vi "BrowseTDMSFile.vi"() -> (1 "No files":bool=TRUE, 3 "Selected traces":string[](array[string]))   [LabVIEW 2018]
uses:
  <vilib>/gmath/statdist.llb/st_Percentiles (scalar).vi
  <vilib>/gmath/NI_Gmath.lvlib
panel:
  in  "Deselect all":bool
  out "ScanCode":i16
  in  "Cancel":bool
  in  "Change file":bool
  in  "Sort":bool
  out "F(z)":cluster{"Data":dbl[], "Data":dbl[]}[](graph)
  in  "Select trace":u16(ring)=65535 items=["C:\\Users\\tweezer_user\\Data\\211221\\data_004.tdms: 58", "C:\\Users\\tweezer_user\\Data\\211221\\data_004.tdms: 0", "C:\\Users\\tweezer_user\\Data\\211221\\data_004.tdms: 2", "C:\\Users\\tweezer_user\\Data\\211221\\data_004.tdms: 30", "C:\\Users\\tweezer_user\\Data\\211221\\data_004.tdms: 44", "C:\\Users\\tweezer_user\\Data\\211221\\data_004.tdms: 55", "C:\\Users\\tweezer_user\\Data\\211221\\data_004.tdms: 41", "C:\\Users\\tweezer_user\\Data\\211221\\data_004.tdms: 22", "C:\\Users\\tweezer_user\\Data\\211221\\data_004.tdms: 48", "C:\\Users\\tweezer_user\\Data\\211221\\data_004.tdms: 21", "C:\\Users\\tweezer_user\\Data\\211221\\data_004.tdms: 24", "C:\\Users\\tweezer_user\\Data\\211221\\data_004.tdms: 54", "C:\\Users\\tweezer_user\\Data\\211221\\data_004.tdms: 1", "C:\\Users\\tweezer_user\\Data\\211221\\data_004.tdms: 3", "C:\\Users\\tweezer_user\\Data\\211221\\data_004.tdms: 11", "C:\\Users\\tweezer_user\\Data\\211221\\data_004.tdms: 39", "C:\\Users\\tweezer_user\\Data\\211221\\data_004.tdms: 25", "C:\\Users\\tweezer_user\\Data\\211221\\data_004.tdms: 45", "C:\\Users\\tweezer_user\\Data\\211221\\data_004.tdms: 37", "C:\\Users\\tweezer_user\\Data\\211221\\data_004.tdms: 38", "C:\\Users\\tweezer_user\\Data\\211221\\data_004.tdms: 43", "C:\\Users\\tweezer_user\\Data\\211221\\data_004.tdms: 50", "C:\\Users\\tweezer_user\\Data\\211221\\data_004.tdms: 10", "C:\\Users\\tweezer_user\\Data\\211221\\data_004.tdms: 42", "C:\\Users\\tweezer_user\\Data\\211221\\data_004.tdms: 4", "C:\\Users\\tweezer_user\\Data\\211221\\data_004.tdms: 23", "C:\\Users\\tweezer_user\\Data\\211221\\data_004.tdms: 34", "C:\\Users\\tweezer_user\\Data\\211221\\data_004.tdms: 32", "C:\\Users\\tweezer_user\\Data\\211221\\data_004.tdms: 28", "C:\\Users\\tweezer_user\\Data\\211221\\data_004.tdms: 31", "C:\\Users\\tweezer_user\\Data\\211221\\data_004.tdms: 33", "C:\\Users\\tweezer_user\\Data\\211221\\data_004.tdms: 35", "C:\\Users\\tweezer_user\\Data\\211221\\data_004.tdms: 6", "C:\\Users\\tweezer_user\\Data\\211221\\data_004.tdms: 18", "C:\\Users\\tweezer_user\\Data\\211221\\data_004.tdms: 19", "C:\\Users\\tweezer_user\\Data\\211221\\data_004.tdms: 36", "C:\\Users\\tweezer_user\\Data\\211221\\data_004.tdms: 29", "C:\\Users\\tweezer_user\\Data\\211221\\data_004.tdms: 53", "C:\\Users\\tweezer_user\\Data\\211221\\data_004.tdms: 57", "C:\\Users\\tweezer_user\\Data\\211221\\data_004.tdms: 20", "C:\\Users\\tweezer_user\\Data\\211221\\data_004.tdms: 7", "C:\\Users\\tweezer_user\\Data\\211221\\data_004.tdms: 56", "C:\\Users\\tweezer_user\\Data\\211221\\data_004.tdms: 47", "C:\\Users\\tweezer_user\\Data\\211221\\data_004.tdms: 51", "C:\\Users\\tweezer_user\\Data\\211221\\data_004.tdms: 49", "C:\\Users\\tweezer_user\\Data\\211221\\data_004.tdms: 9", "C:\\Users\\tweezer_user\\Data\\211221\\data_004.tdms: 8", "C:\\Users\\tweezer_user\\Data\\211221\\data_004.tdms: 12", "C:\\Users\\tweezer_user\\Data\\211221\\data_004.tdms: 5", "C:\\Users\\tweezer_user\\Data\\211221\\data_004.tdms: 14", "C:\\Users\\tweezer_user\\Data\\211221\\data_004.tdms: 40", "C:\\Users\\tweezer_user\\Data\\211221\\data_004.tdms: 27", "C:\\Users\\tweezer_user\\Data\\211221\\data_004.tdms: 46", "C:\\Users\\tweezer_user\\Data\\211221\\data_004.tdms: 13", "C:\\Users\\tweezer_user\\Data\\211221\\data_004.tdms: 16", "C:\\Users\\tweezer_user\\Data\\211221\\data_004.tdms: 15", "C:\\Users\\tweezer_user\\Data\\211221\\data_004.tdms: 52", "C:\\Users\\tweezer_user\\Data\\211221\\data_004.tdms: 17", "C:\\Users\\tweezer_user\\Data\\211221\\data_004.tdms: 26", "C:\\Users\\tweezer_user\\Data\\211221\\data_004.tdms: 473"]
  in  "OK":bool
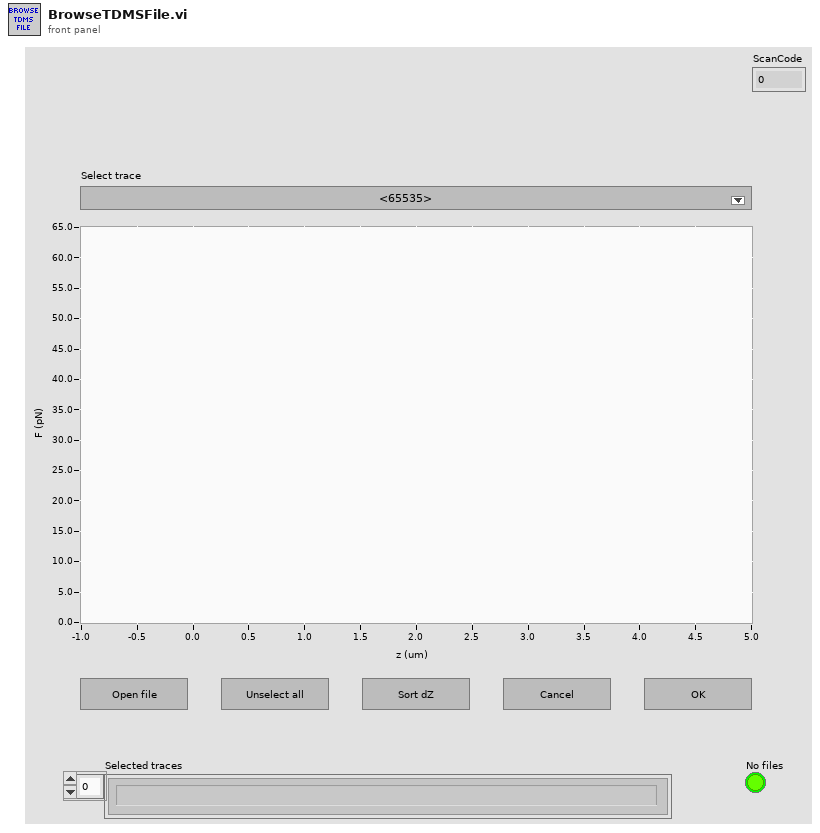
[diagram p1: front panel]
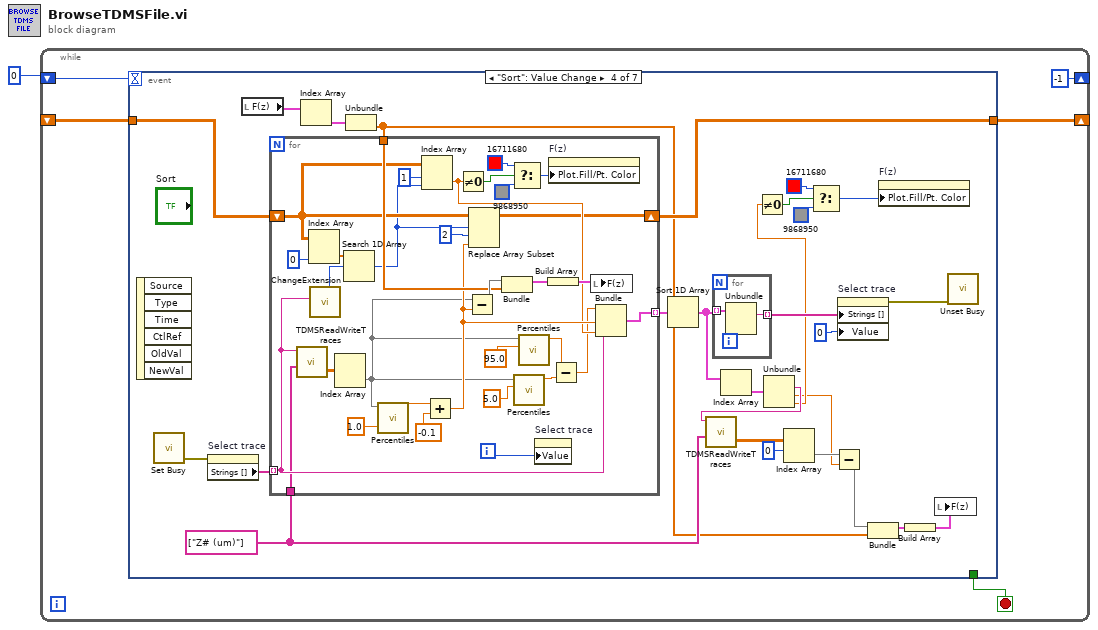
[diagram p0: block diagram]
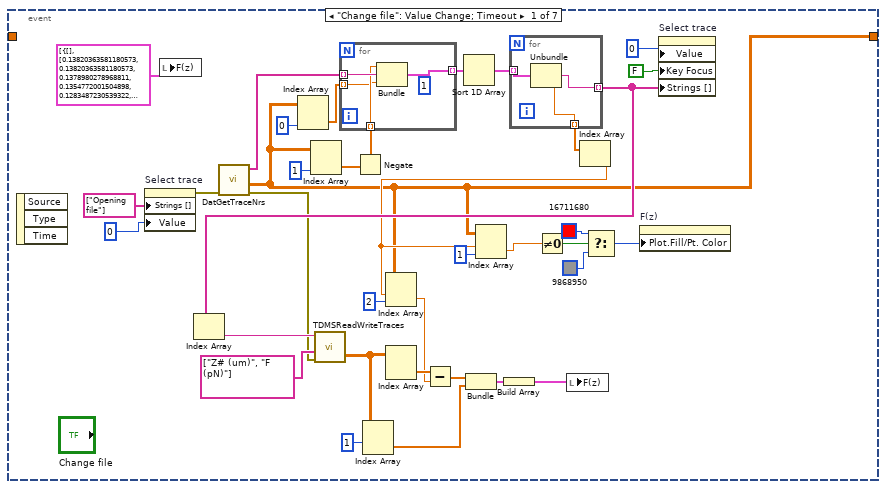
[diagram p2: hidden frame]
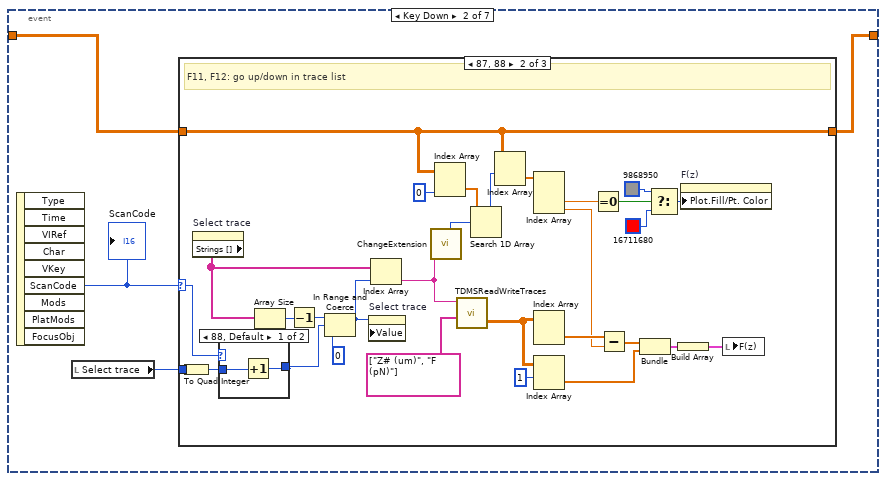
[diagram p3: hidden frame]
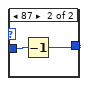
[diagram p5: hidden frame]
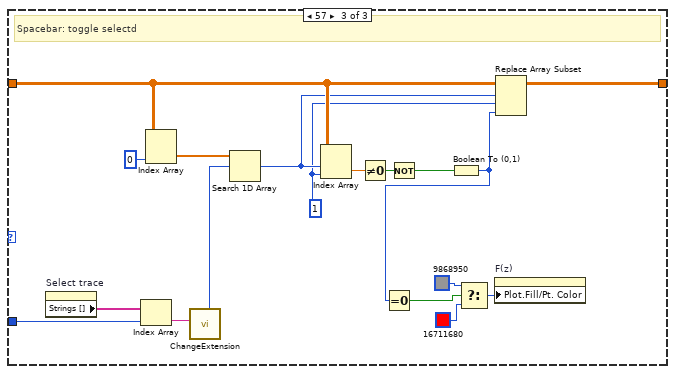
[diagram p6: hidden frame]
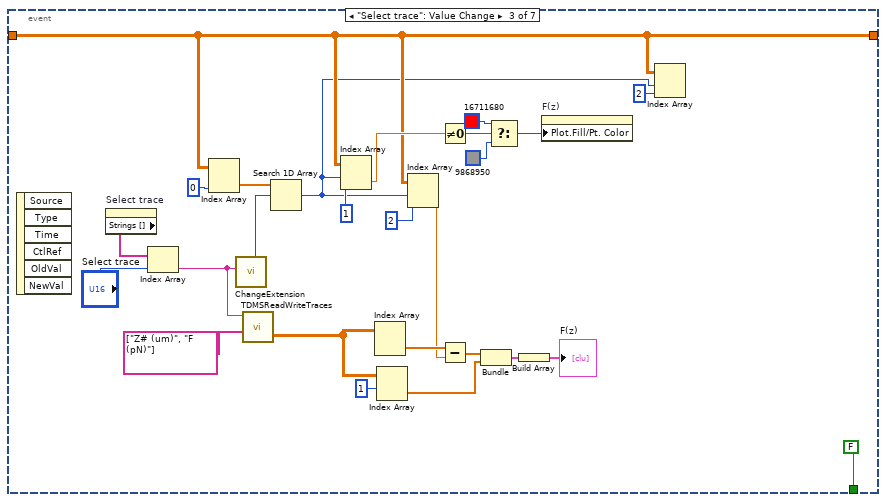
[diagram p7: hidden frame]
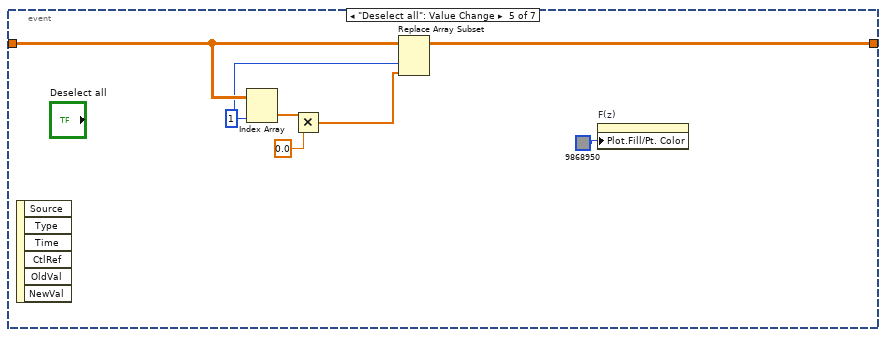
[diagram p8: hidden frame]
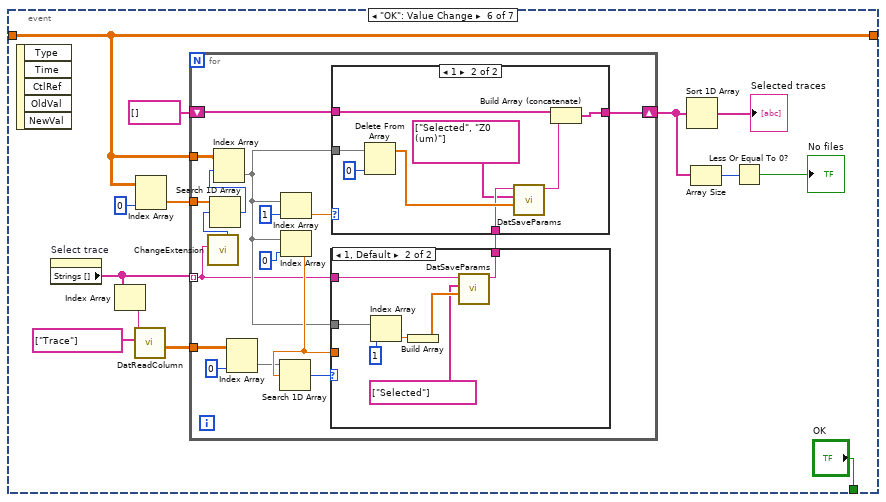
[diagram p9: hidden frame]
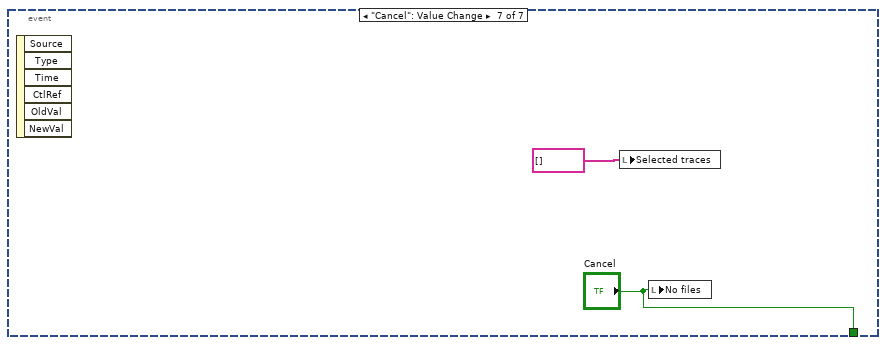
[diagram p12: hidden frame]
diagram:
  n1 = while {
    shift-right: [-1 ("Listbox")] -> _
    shift-left: 0 ("Listbox") -> [w5]
    shift-right: [w2] -> _
    shift-left: _ -> [w3]
    stop <- w6 stop-if-true
    n2 = event shown="[3] \"Sort\": Value Change" {
      selector: _ -> [_ _ _ _ _ _ _]
      dyn-events: _ -> [_ _ _ _ _ _ _]
      timeout: w5 -> [_ _ _ _ _ _ _]
      tunnel: [_ _ FALSE ("stop") _ _ "OK" "Cancel"] -> w6
      tunnel: [w10 w51 w109 w153 w195 w201 _] -> w2
      tunnel: w3 -> [_ w52 w109 w154 w198 w201 _]
      event "Change file": Value Change; Timeout {
        n3 = event-data() -> ()  [unwired: 1 in, 3 out]
        n4 = property on="Select trace" class="Ring (strict)"("Strings []"=string[] ["Opening file"], "Value"=0 ("Top Row")) -> (error out=w23:errorcluster)  [unwired: 2 in, 1 out]
        n5 = local write "F(z)"(cluster{"Data":i32[], "Data":dbl[]}[] [{"Data"=[], "Data"=[0.13820363581180573, 0.13820363581180573, 0.1378980278968811, 0.1354772001504898, 0.1283487230539322, 0.12796370685100555, 0.12760481238365173, 0.12726476788520813, 0.126942977309227, 0.12663885951042175, 0.12635183334350586, 0.12608134746551514, 0.12582682073116302, 0.12558774650096893, 0.1253635585308075, 0.12515376508235931, 0.12495782971382141, 0.1247752457857132, 0.12460550665855408, 0.12444813549518585, 0.12430262565612793, 0.1241685003042221, 0.12404527515172958, 0.12393248826265335, 0.12382965534925461, 0.12373632192611694, 0.12365201860666275, 0.12357629835605621, 0.12350869178771973, 0.12344875186681747, 0.12339602410793304, 0.12335006892681122, 0.12331042438745499, 0.12327665835618973, 0.12324832379817963, 0.12322498112916946, 0.12320617586374283, 0.1231914833188057, 0.12318044900894165, 0.12317264080047607, 0.12316761910915375, 0.12316494435071945, 0.12316489964723587, 0.12408066540956497, 0.12665148079395294, 0.13009892404079437, 0.13340164721012115, 0.1366782933473587, 0.1401367038488388, 0.1436801254749298, 0.14730530977249146, 0.15101973712444305, 0.15482020378112793, 0.15873165428638458, 0.16275079548358917, 0.16688737273216248, 0.17111752927303314, 0.17530791461467743, 0.17975105345249176, 0.1843348741531372, 0.1890215128660202, 0.19384075701236725, 0.19893240928649902, 0.20381732285022736, 0.20893964171409607, 0.21432308852672577, 0.21960188448429108, 0.22516034543514252, 0.23087568581104279, 0.2368132770061493, 0.2428968846797943, 0.24884368479251862, 0.25512930750846863, 0.26159971952438354, 0.268232524394989, 0.2750486135482788, 0.2820947766304016, 0.2891634702682495, 0.296439528465271, 0.3039502501487732, 0.3116407096385956, 0.31944137811660767, 0.32760921120643616, 0.3358848989009857, 0.34432253241539, 0.3531827926635742, 0.3622758090496063, 0.3714924454689026, 0.3809875249862671, 0.39067110419273376, 0.4001978039741516, 0.4104802906513214, 0.42095404863357544, 0.43167173862457275, 0.44273218512535095, 0.45405450463294983, 0.4653382897377014, 0.47709932923316956, 0.4893254041671753, 0.5018249154090881, 0.5145537853240967, 0.5275917649269104, 0.541254997253418, 0.5551921725273132, 0.5689001679420471, 0.5834644436836243, 0.5981636643409729, 0.6131883263587952, 0.6288307309150696, 0.645302414894104, 0.6615437865257263, 0.6788241863250732, 0.6965782642364502, 0.7143076658248901, 0.7322126030921936, 0.7507462501525879, 0.7696933746337891, 0.7891842722892761, 0.8094238638877869, 0.8305338025093079, 0.8516679406166077, 0.873047947883606, 0.8949730396270752, 0.9177820086479187, 0.941853940486908, 0.9660325646400452, 0.9906901717185974, 1.0159856081008911, 1.041857361793518, 1.0686113834381104, 1.0960968732833862, 1.124282717704773, 1.1531327962875366, 1.1826114654541016, 1.2131890058517456, 1.244091272354126, 1.2758408784866333, 1.308860421180725, 1.3426004648208618, 1.377321481704712, 1.4129451513290405, 1.4491798877716064, 1.4859497547149658, 1.5242410898208618, 1.5638980865478516, 1.6039670705795288, 1.6451531648635864, 1.6887091398239136, 1.731339931488037, 1.7758506536483765, 1.8221782445907593, 1.8698104619979858, 1.9181337356567383, 1.9674079418182373, 2.0180675983428955, 2.0700340270996094, 2.12361741065979, 2.1799402236938477, 2.235238552093506, 2.2942440509796143, 2.3544530868530273, 2.413398265838623, 2.4763426780700684, 2.540114641189575, 2.6063880920410156, 2.674560785293579, 2.743506908416748, 2.8154006004333496, 2.888751268386841, 2.9644055366516113, 3.0424892902374268, 3.122440814971924, 3.2058236598968506, 3.287494659423828, 3.371485471725464, 3.4608986377716064, 3.5549445152282715, 3.6497061252593994, 3.745452880859375, 3.840704917907715, 3.9366137981414795, 4.041317462921143, 4.151824474334717, 4.260120391845703, 4.369058609008789, 4.484458923339844, 4.602372646331787, 4.723849296569824, 4.849534034729004, 4.97871732711792, 5.11023473739624, 5.247971534729004, 5.384191513061523, 5.524545192718506, 5.672408580780029, 5.825640678405762, 5.974457263946533, 6.13252067565918, 6.29857873916626, 6.468328952789307, 6.63914155960083, 6.8164191246032715, 6.998229503631592, 7.18559455871582, 7.379547595977783, 7.577399730682373, 7.778872013092041, 7.987000465393066, 8.203492164611816, 8.42825698852539, 8.657670974731445, 8.88441276550293, 9.119434356689453, 9.369271278381348, 9.631810188293457, 9.883063316345215, 10.155534744262695, 10.431879997253418, 10.704452514648438, 10.995787620544434, 11.301190376281738, 11.602027893066406, 11.912508010864258, 12.24520206451416, 12.577718734741211, 12.921031951904297, 13.28329086303711, 13.65456771850586, 14.021306037902832, 14.397754669189453, 14.797367095947266, 15.205953598022461, 15.621662139892578, 16.054304122924805, 16.50411033630371, 16.959596633911133, 17.4282169342041, 17.912626266479492, 18.40574073791504, 18.916988372802734, 19.45334815979004, 19.999784469604492, 20.54841423034668, 21.119876861572266, 21.71088981628418, 22.32358741760254, 22.962291717529297, 23.62326431274414, 24.269819259643555, 24.959508895874023, 25.66047477722168, 26.40703582763672, 27.107582092285156, 27.192604064941406, 27.273927688598633, 27.35161018371582, 27.425710678100586, 27.49629020690918, 27.563413619995117, 27.62714958190918, 27.687564849853516, 27.744731903076172, 27.798725128173828, 27.84961700439453, 27.897485733032227, 27.942411422729492, 27.984472274780273, 28.023752212524414, 28.060335159301758, 28.094303131103516, 28.125743865966797, 28.154747009277344, 28.181396484375, 28.205785751342773, 28.228002548217773, 28.248138427734375, 28.266286849975586, 28.28253936767578, 28.2969913482666, 28.30973243713379, 28.32086181640625, 28.330472946166992, 28.338659286499023, 28.345518112182617, 28.351146697998047, 28.355640411376953, 28.359094619750977, 28.36160659790039, 28.36327362060547, 28.364192962646484, 28.363798141479492, 28.108924865722656, 27.453271865844727, 26.65618133544922, 25.92983055114746, 25.214139938354492, 24.494150161743164, 23.814538955688477, 23.16864585876465, 22.546876907348633, 21.9448184967041, 21.345447540283203, 20.75084686279297, 20.185226440429688, 19.650880813598633, 19.09626579284668, 18.594301223754883, 18.099639892578125, 17.606752395629883, 17.126239776611328, 16.66429901123047, 16.221187591552734, 15.787714004516602, 15.362269401550293, 14.949151992797852, 14.556093215942383, 14.165535926818848, 13.781983375549316, 13.411600112915039, 13.05821704864502, 12.710689544677734, 12.370074272155762, 12.04362964630127, 11.72891616821289, 11.405869483947754, 11.109034538269043, 10.817221641540527, 10.53183364868164, 10.25683307647705, 9.981552124023438, 9.71689224243164, 9.462623596191406, 9.215733528137207, 8.97307014465332, 8.737778663635254, 8.504226684570312, 8.27858829498291, 8.063911437988281, 7.858738422393799, 7.652857780456543, 7.456949710845947, 7.260039806365967, 7.062727928161621, 6.8852219581604, 6.707188606262207, 6.533257007598877, 6.363514423370361, 6.196928977966309, 6.032388687133789, 5.874703884124756, 5.722533226013184, 5.576818466186523, 5.43751859664917, 5.296698093414307, 5.160645008087158, 5.029038906097412, 4.899881362915039, 4.771241664886475, 4.649013996124268, 4.529282093048096, 4.413956165313721, 4.301394462585449, 4.185991287231445, 4.0807785987854, 3.97784686088562, 3.876406669616699, 3.7768642902374268, 3.678968667984009, 3.5860061645507812, 3.4950578212738037, 3.4059789180755615, 3.3189303874969482, 3.231165647506714, 3.1516504287719727, 3.072159767150879, 2.9924099445343018, 2.9165806770324707, 2.843553066253662, 2.7714359760284424, 2.7004895210266113, 2.631819486618042, 2.566622018814087, 2.500638008117676, 2.437282085418701, 2.3751180171966553, 2.3141775131225586, 2.2577991485595703, 2.1997828483581543, 2.1441314220428467, 2.0905234813690186, 2.0375893115997314, 1.9846081733703613, 1.9357779026031494, 1.8867290019989014, 1.8384720087051392, 1.7935200929641724, 1.7484320402145386, 1.7043356895446777, 1.661389708518982, 1.6195507049560547, 1.5787100791931152, 1.5393437147140503, 1.500795602798462, 1.4630988836288452, 1.426209568977356, 1.3899059295654297, 1.3552272319793701, 1.3215932846069336, 1.2886830568313599, 1.256393551826477, 1.2249362468719482, 1.1946345567703247, 1.1640089750289917, 1.1342456340789795, 1.1066683530807495, 1.0792484283447266, 1.052013635635376, 1.0255601406097412, 0.9999175071716309, 0.9748290777206421, 0.9509499073028564, 0.9273965358734131, 0.9039201140403748, 0.8808199763298035, 0.8588014245033264, 0.8371475338935852, 0.8165111541748047, 0.7966588735580444, 0.7771881818771362, 0.7577195167541504, 0.7387968301773071, 0.7206172347068787, 0.7028306722640991, 0.6851621270179749, 0.6681071519851685, 0.6514108180999756, 0.6354106664657593, 0.6196495890617371, 0.6036196351051331, 0.5889309048652649, 0.5744688510894775, 0.5602098107337952, 0.5462936162948608, 0.5328689217567444, 0.519416093826294, 0.5065906643867493, 0.49413758516311646, 0.4818674325942993, 0.4698854982852936, 0.4580205976963043, 0.4466813802719116, 0.435754656791687, 0.4250485301017761, 0.4145328402519226, 0.40424683690071106, 0.39417997002601624, 0.3844664692878723, 0.3751589059829712, 0.3657279312610626, 0.3566521406173706, 0.3478308320045471, 0.339187353849411, 0.3307023346424103, 0.32244783639907837, 0.31454113125801086, 0.3068597614765167, 0.2993113100528717, 0.2918766438961029, 0.2844787538051605, 0.27748575806617737, 0.2707583010196686, 0.26413148641586304, 0.2576119303703308, 0.25112348794937134, 0.2448214888572693, 0.2387808859348297, 0.23297420144081116, 0.22715920209884644, 0.22166672348976135, 0.21626408398151398, 0.21090243756771088, 0.20566461980342865, 0.2006448209285736, 0.1956656128168106, 0.19083058834075928, 0.18618997931480408, 0.18170233070850372, 0.1771688163280487, 0.17275111377239227, 0.16845916211605072, 0.16429205238819122, 0.16027286648750305, 0.15627284348011017, 0.1524406224489212, 0.14844897389411926, 0.14537310600280762, 0.14513526856899261, 0.14490433037281036, 0.1446801722049713, 0.1444626748561859, 0.14425170421600342, 0.14404717087745667, 0.14384892582893372, 0.1436568945646286, 0.14347092807292938, 0.1432909220457077, 0.1431167721748352, 0.14294837415218353, 0.14278562366962433, 0.14262838661670685, 0.14247657358646393, 0.1423300802707672, 0.14218880236148834, 0.14205263555049896, 0.14192146062850952, 0.14179520308971405, 0.141673743724823, 0.1415569931268692, 0.1414448320865631, 0.14133718609809875, 0.14123395085334778, 0.14113502204418182, 0.14104029536247253, 0.14094969630241394, 0.14086312055587769, 0.1407804638147354, 0.14070165157318115, 0.14062656462192535, 0.14055512845516205, 0.14048723876476288, 0.14042282104492188, 0.1403617560863495, 0.14030396938323975, 0.1402493715286255, 0.14019787311553955, 0.14014936983585358, 0.1401037722826004, 0.14006102085113525, 0.14002098143100739, 0.13998359441757202, 0.1399487555027008, 0.13991639018058777, 0.13988640904426575, 0.13985870778560638, 0.13983319699764252, 0.13980981707572937, 0.1397884488105774, 0.13976901769638062, 0.13975143432617188, 0.1397356241941452, 0.13972148299217224, 0.13970892131328583, 0.13969786465168, 0.13968820869922638, 0.1396798938512802, 0.13967280089855194, 0.1396668702363968, 0.1396619975566864, 0.1396581083536148, 0.13965511322021484, 0.13965290784835815, 0.13965141773223877, 0.13965056836605072, 0.13965025544166565, 0.1404738873243332, 0.14295253157615662, 0.14680111408233643, 0.1505328267812729, 0.15433314442634583, 0.1582556813955307, 0.16225314140319824, 0.1663271188735962, 0.17052745819091797, 0.17483928799629211, 0.17925673723220825, 0.18379244208335876, 0.18845663964748383, 0.19324597716331482, 0.19808430969715118, 0.20306238532066345, 0.20828750729560852, 0.21372802555561066, 0.21891967952251434, 0.22443637251853943, 0.23011063039302826, 0.2359151542186737, 0.2419096678495407, 0.24810093641281128, 0.25437018275260925, 0.2608209252357483, 0.26743221282958984, 0.2740837037563324, 0.28103750944137573, 0.28832897543907166, 0.2957537770271301, 0.3031705319881439, 0.31062212586402893, 0.3184690475463867, 0.3265407979488373, 0.3349866271018982, 0.34377002716064453, 0.3521841764450073, 0.36087876558303833, 0.37003475427627563, 0.379533976316452, 0.389178991317749, 0.3991386592388153, 0.4093271791934967, 0.4196397662162781, 0.4301832914352417, 0.44114720821380615, 0.45235514640808105, 0.46388524770736694, 0.47590339183807373, 0.48817381262779236, 0.5001714825630188, 0.5128669142723083, 0.5258751511573792, 0.5394296646118164, 0.5534142255783081, 0.5670239329338074, 0.5814993381500244, 0.5963174104690552, 0.6114774942398071, 0.627088725566864, 0.6431040167808533, 0.6594688892364502, 0.6763340830802917, 0.6936191320419312, 0.7111948132514954, 0.7292730808258057, 0.7484663128852844, 0.7681370973587036, 0.7876899838447571, 0.8069140315055847, 0.8273855447769165, 0.8483879566192627, 0.87064528465271, 0.8937667608261108, 0.9157674908638, 0.9390804171562195, 0.9628303647041321, 0.9873177409172058, 1.0129517316818237, 1.0397191047668457, 1.0651978254318237, 1.0922280550003052, 1.1206347942352295, 1.14925217628479, 1.1786895990371704, 1.2089424133300781, 1.2402781248092651, 1.2723357677459717, 1.3045451641082764, 1.3380173444747925, 1.3723875284194946, 1.4078353643417358, 1.4444127082824707, 1.481903314590454, 1.519201397895813, 1.558168649673462, 1.5984965562820435, 1.6399141550064087, 1.6835541725158691, 1.7262741327285767, 1.7705788612365723, 1.8163195848464966, 1.8626331090927124, 1.9106162786483765, 1.9612172842025757, 2.013096570968628, 2.064939498901367, 2.1162948608398438, 2.1709985733032227, 2.227315902709961, 2.2851991653442383, 2.3445701599121094, 2.405320882797241, 2.470532178878784, 2.5336344242095947, 2.5976805686950684, 2.6655802726745605, 2.7353603839874268, 2.8051135540008545, 2.879950523376465, 2.956644296646118, 3.0310230255126953, 3.1104393005371094, 3.1925745010375977, 3.2760515213012695, 3.361126661300659, 3.4490272998809814, 3.538938522338867, 3.6318559646606445, 3.7271268367767334, 3.8252601623535156, 3.927900552749634, 4.02937650680542, 4.133993625640869, 4.242278575897217, 4.354728698730469, 4.473111629486084, 4.588019847869873, 4.708067893981934, 4.832813262939453, 4.959743022918701, 5.090849876403809, 5.2276930809021, 5.367144584655762, 5.508208274841309, 5.6519060134887695, 5.801891326904297, 5.956840991973877, 6.1145124435424805, 6.277387619018555, 6.451018333435059, 6.62131929397583, 6.794903755187988, 6.974320888519287, 7.161947727203369, 7.360052108764648, 7.554330348968506, 7.755161762237549, 7.961829662322998, 8.172811508178711, 8.393034934997559, 8.614129066467285, 8.851072311401367, 9.099882125854492, 9.34743595123291, 9.587959289550781, 9.845237731933594, 10.114744186401367, 10.391414642333984, 10.672096252441406, 10.959001541137695, 11.255366325378418, 11.56225872039795, 11.8775053024292, 12.1961030960083, 12.527969360351562, 12.87659740447998, 13.232915878295898, 13.591902732849121, 13.963973045349121, 14.34652042388916, 14.74950885772705, 15.157404899597168, 15.55984115600586, 16.00151252746582, 16.43935775756836, 16.900432586669922, 17.37667465209961, 17.843921661376953, 18.33938980102539, 18.84848976135254, 19.374143600463867, 19.91344451904297, 20.458410263061523, 21.035266876220703, 21.635311126708984, 22.246536254882812, 22.86618995666504, 23.508785247802734, 24.177562713623047, 24.8514404296875, 25.54566764831543, 26.28206443786621, 27.10145378112793, 27.210445404052734, 27.292709350585938, 27.371305465698242, 27.4462947845459, 27.517738342285156, 27.5856990814209, 27.650245666503906, 27.71144676208496, 27.769372940063477, 27.824098587036133, 27.875696182250977, 27.924245834350586, 27.969825744628906, 28.012516021728516, 28.052398681640625, 28.089557647705078, 28.12407684326172, 28.15604591369629, 28.185548782348633, 28.212675094604492, 28.237516403198242, 28.260160446166992, 28.28070068359375, 28.29922866821289, 28.315839767456055, 28.330623626708984, 28.343677520751953, 28.3550968170166, 28.364974975585938, 28.373409271240234, 28.380495071411133, 28.386327743530273, 28.391006469726562, 28.39462661743164, 28.39728546142578, 28.39908218383789, 28.40011215209961, 28.40047264099121, 28.176712036132812, 27.567598342895508, 26.74456787109375, 26.02675437927246, 25.331581115722656, 24.625301361083984, 23.935752868652344, 23.270889282226562, 22.627761840820312, 22.008010864257812, 21.424182891845703, 20.85088348388672, 20.282140731811523, 19.728761672973633, 19.180891036987305, 18.64856719970703, 18.14957618713379, 17.678686141967773, 17.201255798339844, 16.736671447753906, 16.28534698486328, 15.847111701965332, 15.42111873626709, 15.005548477172852, 14.60929012298584, 14.212642669677734, 13.822290420532227, 13.454268455505371, 13.100285530090332, 12.758034706115723, 12.421067237854004, 12.089723587036133, 11.76894474029541, 11.449254035949707, 11.143107414245605, 10.84855842590332, 10.564229965209961, 10.292014122009277, 10.02628231048584, 9.7589111328125, 9.497990608215332, 9.24967098236084, 9.00622844696045, 8.770873069763184, 8.54104232788086, 8.317278861999512, 8.100481986999512, 7.887633323669434, 7.680600643157959, 7.481308460235596, 7.287881851196289, 7.09689474105835, 6.912325382232666, 6.732483863830566, 6.557768821716309, 6.388072490692139, 6.222366809844971, 6.056153774261475, 5.899376392364502, 5.747296333312988, 5.5975565910339355, 5.457229137420654, 5.319812297821045, 5.183464050292969, 5.0478105545043945, 4.913556098937988, 4.7820820808410645, 4.662775039672852, 4.546417713165283, 4.430275917053223, 4.315897464752197, 4.205315589904785, 4.097395896911621, 3.992088556289673, 3.8899497985839844, 3.791670560836792, 3.6945459842681885, 3.5975446701049805, 3.5053722858428955, 3.418710708618164, 3.331511974334717, 3.246521472930908, 3.161881923675537, 3.0808229446411133, 3.0048415660858154, 2.9281411170959473, 2.8540608882904053, 2.7817068099975586, 2.710829257965088, 2.6414480209350586, 2.573183059692383, 2.5067813396453857, 2.444240093231201, 2.3844492435455322, 2.3243162631988525, 2.2652533054351807, 2.2084155082702637, 2.152742862701416, 2.097804069519043, 2.0446836948394775, 1.9932688474655151, 1.9430584907531738, 1.8940881490707397, 1.8463551998138428, 1.7993099689483643, 1.754496693611145, 1.7106740474700928, 1.6676170825958252, 1.6255496740341187, 1.584224820137024, 1.5447214841842651, 1.506205439567566, 1.4683912992477417, 1.4314963817596436, 1.3954071998596191, 1.3607169389724731, 1.3263353109359741, 1.2924476861953735, 1.2608832120895386, 1.2293668985366821, 1.1985576152801514, 1.1685947179794312, 1.1393409967422485, 1.110318660736084, 1.0833029747009277, 1.0563404560089111, 1.0296366214752197, 1.003867506980896, 0.9780988097190857, 0.9536804556846619, 0.930267870426178, 0.9074224233627319, 0.8848013281822205, 0.862708568572998, 0.8411343097686768, 0.8201403617858887, 0.7997604012489319, 0.7799765467643738, 0.7605317831039429, 0.7415838241577148, 0.7231556177139282, 0.7051433324813843, 0.6872482895851135, 0.6706206202507019, 0.6540273427963257, 0.6375616192817688, 0.6216949224472046, 0.6062119007110596, 0.5911306738853455, 0.5766394138336182, 0.5625021457672119, 0.548316478729248, 0.5343603491783142, 0.5211761593818665, 0.5084199905395508, 0.49588483572006226, 0.4836081266403198, 0.47162121534347534, 0.45993572473526, 0.4484090507030487, 0.4370848834514618, 0.4263474643230438, 0.41597920656204224, 0.4057176411151886, 0.3956356346607208, 0.38584861159324646, 0.37624144554138184, 0.3670654296875, 0.35797417163848877, 0.3490314781665802, 0.34045088291168213, 0.3320196568965912, 0.32367876172065735, 0.3155428469181061, 0.30772659182548523, 0.30028825998306274, 0.2929779589176178, 0.28559842705726624, 0.27851149439811707, 0.27175062894821167, 0.2648177146911621, 0.2584708034992218, 0.2521646320819855, 0.24592699110507965, 0.23984010517597198, 0.23374046385288239, 0.22808296978473663, 0.22253361344337463, 0.21703961491584778, 0.21167171001434326, 0.2064555436372757, 0.2013399600982666, 0.1962956190109253, 0.19141532480716705, 0.18681776523590088, 0.18222449719905853, 0.17773021757602692, 0.17335669696331024, 0.16903990507125854, 0.164662703871727, 0.16084024310112, 0.15693038702011108, 0.15302087366580963, 0.1491761952638626, 0.1450546383857727, 0.14497064054012299, 0.14497064054012299, 0.14497064054012299, 0.14497064054012299, 0.14497064054012299, 0.14497064054012299, 0.14497064054012299, 0.14497064054012299, 0.14497064054012299, 0.14497064054012299, 0.14497064054012299, 0.14497064054012299, 0.14497064054012299, 0.14497064054012299, 0.14497064054012299, 0.14497064054012299, 0.14497064054012299, 0.14497064054012299, 0.14497064054012299, 0.14497064054012299, 0.14497064054012299, 0.14497064054012299, 0.14497064054012299]}] ("F(z)")) -> ()
        n6 = call "DatGetTraceNrs.vi"("error in (no error)"=w23) -> ("error out"=w7:errorcluster, "Par values"=w10:dbl[][], "All Traces"=w15:string[])  [unwired: 6 in, 2 out]
        n7 = Index Array(array=w10, index (col)=0 ("disabled index (col)")) -> (element=w9:dbl[])  [unwired: 1 in]
        n8 = Index Array(array=w10, index (col)=1 ("disabled index (col)")) -> (element=w18:dbl[])  [unwired: 1 in]
        n9 = Negate(x=w18) -> (-x=w17:dbl[])
        n10 = for {
          tunnel: w15 -> [w49] mode=indexing
          tunnel: [w48] -> w20 mode=indexing
          tunnel: w17 -> [w47] mode=indexing
          tunnel: w9 -> [w46] mode=indexing
          (unwired) 1 ("index")
          n11 = Bundle("element"=w47, w49, "element"=w46) -> (w48:cluster{"element":dbl, string, "element":dbl})  [unwired: 1 in]
        }
        n12 = Sort 1D Array(array=w20) -> (sorted array=w16:cluster{"element":dbl, string, "element":dbl}[])
        n13 = for {
          tunnel: w16 -> [w45] mode=indexing
          tunnel: [w44] -> w14 mode=indexing
          tunnel: [w43] -> w13 mode=indexing
          n14 = Unbundle(w45) -> (w44:string, "element"=w43:dbl)  [unwired: 1 out]
        }
        n15 = Index Array(array=w14) -> (element=w27:string)  [unwired: 1 in]
        n16 = call "TDMSReadWriteTraces.vi"("error in (no error)"=w7, "Channels in"=string[] ["Z# (um)", "F (pN)"], "tracename"=w27) -> ("Data out"=w41:dbl[][])  [unwired: 3 in, 5 out]
        n17 = Index Array(array=w41, index (row)=1) -> (element=w40:dbl[])  [unwired: 1 in]
        n18 = Index Array(array=w41) -> (element=w38:dbl[])  [unwired: 2 in]
        n19 = Index Array(array=w13) -> (element=w12:dbl)  [unwired: 1 in]
        n20 = Index Array(array=w10, index (row)=w12, index (col)=2 ("disabled index (col)")) -> (element=w25:dbl)
        n21 = Subtract(x=w38, y=w25) -> (x-y=w37:dbl[])
        n22 = Bundle(w37, "Data out"=w40) -> (w26:cluster{dbl[], "Data out":dbl[]})  [unwired: 1 in]
        n23 = Index Array(array=w10, index (row)=w12, index (col)=1 ("disabled index (col)")) -> (element=w30:dbl)
        n24 = Build Array(w26) -> (w34:cluster{dbl[], "Data out":dbl[]}[])
        n25 = Not Equal To 0?(x=w30) -> (x != 0?=w31:bool)
        n26 = local write "F(z)"(w34) -> ()
        n27 = Select(t=u32 16711680, s=w31, f=u32 9868950) -> (s? t:f=w29:u32)
        n28 = property on="F(z)" class="XYGraph (strict)"("Plot.Fill/Pt. Color"=w29) -> ()  [unwired: 2 in, 2 out]
        n29 = property on="Select trace" class="Ring (strict)"("Value"=0 ("Top Row"), "Key Focus"=FALSE, "Strings []"=w14) -> ()  [unwired: 2 in, 2 out]
      }
      event Key Down {
        n30 = event-data() -> ("ScanCode"=w53:i16)  [unwired: 1 in, 8 out]
        "ScanCode" <- w53
        n31 = local read "Select trace"() -> (w50:u16)
        n32 = case shown="87, 88" w53 {
          selector: w53 -> [_ w62 _]
          tunnel: w52 -> [w54 w59 w99]
          tunnel: [w54 w59 w104] -> w51
          tunnel: w50 -> [_ w63 w95]
          frame 0, Default {
          }
          frame 87, 88 {
            # "F11, F12: go up/down in trace list"
            n33 = To Quad Integer(1:w63) -> (0:w61:i64)
            n34 = property on="Select trace" class="Ring (strict)"() -> ("Strings []"=w73:string[])  [unwired: 2 in, 2 out]
            n35 = case shown="88, Default" w62 {
              tunnel: [w86 w88] -> w81
              tunnel: w61 -> [w85 w87]
              frame 88, Default {
                n36 = Increment(x=w85) -> (x+1=w86:i64)
              }
              frame 87 {
                n37 = Decrement(x=w87) -> (x-1=w88:i64)
              }
            }
            n38 = Array Size(array=w73) -> (size(s)=w84:i32)
            n39 = Decrement(x=w84) -> (x-1=w83:i32)
            n40 = In Range and Coerce(upper limit=w83, x=w81, lower limit=i64 0) -> (coerced(x)=w71:i64)  [unwired: 1 out]
            n41 = property on="Select trace" class="Ring (strict)"("Value"=w71) -> ()  [unwired: 2 in, 2 out]
            n42 = Index Array(array=w73, index=w71) -> (element=w60:string)
            n43 = call "ChangeExtension.vi"("file in"=w60) -> ("Tracenr"=w56:i32)  [unwired: 4 in, 4 out]
            n44 = Index Array(array=w59, index (col)=0 ("disabled index (col)")) -> (element=w57:dbl[])  [unwired: 1 in]
            n45 = call "TDMSReadWriteTraces.vi"("Channels in"=string[] ["Z# (um)", "F (pN)"], "tracename"=w60) -> ("Data out"=w79:dbl[][])  [unwired: 4 in, 5 out]
            n46 = Search 1D Array(1D array=w57, element=w56) -> (index of element=w55:i32)  [unwired: 1 in]
            n47 = Index Array(array=w59, index (row)=w55) -> (element=w70:dbl[])  [unwired: 1 in]
            n48 = Index Array(array=w70) -> (element #2=w64:dbl, element #3=w69:dbl)  [unwired: 3 in, 1 out]
            n49 = Index Array(array=w79) -> (element=w75:dbl[])  [unwired: 2 in]
            n50 = Index Array(array=w79, index (row)=1) -> (element=w78:dbl[])  [unwired: 1 in]
            n51 = Equal To 0?(x=w64) -> (x = 0?=w68:bool)
            n52 = Subtract(x=w75, y=w69) -> (x-y=w74:dbl[])
            n53 = Bundle(w74, "Data out"=w78) -> (w77:cluster{dbl[], "Data out":dbl[]})  [unwired: 1 in]
            n54 = Select(t=u32 9868950, s=w68, f=u32 16711680) -> (s? t:f=w65:u32)
            n55 = Build Array(w77) -> (w72:cluster{dbl[], "Data out":dbl[]}[])
            n56 = property on="F(z)" class="XYGraph (strict)"("Plot.Fill/Pt. Color"=w65) -> ()  [unwired: 2 in, 2 out]
            n57 = local write "F(z)"(w72) -> ()
          }
          frame 57 {
            w91 = 1 ("index (row)")
            # "Spacebar: toggle selectd"
            n58 = property on="Select trace" class="Ring (strict)"() -> ("Strings []"=w97:string[])  [unwired: 2 in, 2 out]
            n59 = Index Array(array=w97, index=w95) -> (element=w96:string)
            n60 = Index Array(array=w99, index (col)=0 ("index (row)")) -> (element=w106:dbl[])  [unwired: 1 in]
            n61 = call "ChangeExtension.vi"("file in"=w96) -> ("Tracenr"=w105:i32)  [unwired: 4 in, 4 out]
            n62 = Search 1D Array(1D array=w106, element=w105) -> (index of element=w98:i32)  [unwired: 1 in]
            n63 = Index Array(array=w99, index (row)=w98, index (col)=w91) -> (element=w94:dbl)
            n64 = Not Equal To 0?(x=w94) -> (x != 0?=w93:bool)
            n65 = Not(x=w93) -> (.not. x?=w92:bool)
            n66 = Boolean To (0,1)(Boolean=w92) -> (0, 1=w89:i16)
            n67 = Equal To 0?(x=w89) -> (x = 0?=w90:bool)
            n68 = Select(t=u32 9868950, s=w90, f=u32 16711680) -> (s? t:f=w101:u32)
            n69 = property on="F(z)" class="XYGraph (strict)"("Plot.Fill/Pt. Color"=w101) -> ()  [unwired: 2 in, 2 out]
            n70 = Replace Array Subset(array=w99, new element=w89, index (row)=w98, index (col)=w91) -> (w104:dbl[][])
          }
        }
      }
      event "Select trace": Value Change {
        n71 = event-data() -> ()  [unwired: 1 in, 6 out]
        n72 = property on="Select trace" class="Ring (strict)"() -> ("Strings []"=w131:string[])  [unwired: 2 in, 2 out]
        n73 = Index Array(array=w131, index="Select trace") -> (element=w124:string)
        n74 = Index Array(array=w109, index (col)=0 ("index (row)")) -> (element=w123:dbl[])  [unwired: 1 in]
        n75 = call "ChangeExtension.vi"("file in"=w124) -> ("Tracenr"=w122:i32)  [unwired: 4 in, 4 out]
        n76 = call "TDMSReadWriteTraces.vi"("Channels in"=string[] ["Z# (um)", "F (pN)"], "tracename"=w124) -> ("Data out"=w129:dbl[][])  [unwired: 4 in, 5 out]
        n77 = Search 1D Array(1D array=w123, element=w122) -> (index of element=w108:i32)  [unwired: 1 in]
        n78 = Index Array(array=w109, index (row)=w108, index (col)=1 ("index (row)")) -> (element=w117:dbl)
        n79 = Index Array(array=w129) -> (element=w116:dbl[])  [unwired: 2 in]
        n80 = Index Array(array=w129, index (row)=1) -> (element=w128:dbl[])  [unwired: 1 in]
        n81 = Index Array(array=w109, index (row)=w108, index (col)=2 ("disabled index (row)")) -> (element=w114:dbl)
        n82 = Not Equal To 0?(x=w117) -> (x != 0?=w118:bool)
        n83 = Subtract(x=w116, y=w114) -> (x-y=w115:dbl[])
        n84 = Bundle(w115, "Data out"=w128) -> (w127:cluster{dbl[], "Data out":dbl[]})  [unwired: 1 in]
        n85 = Select(t=u32 16711680, s=w118, f=u32 9868950) -> (s? t:f=w119:u32)
        n86 = Build Array(w127) -> (→"F(z)":cluster{dbl[], "Data out":dbl[]}[])
        n87 = property on="F(z)" class="XYGraph (strict)"("Plot.Fill/Pt. Color"=w119) -> ()  [unwired: 2 in, 2 out]
        n88 = Index Array(array=w109, index (row)=w108, index (col)=2 ("disabled index (col)")) -> ()  [unwired: 1 out]
      }
      event "Sort": Value Change {
        w149 = string[] ["Z# (um)"]
        n89 = event-data() -> ()  [unwired: 1 in, 6 out]
        n90 = call <vilib>:"Set Busy.vi"() -> ("error out"=w158:errorcluster)  [unwired: 10 in, 1 out]
        n91 = property on="Select trace" class="Ring (strict)"(error in=w158) -> ("Strings []"=w152:string[])  [unwired: 1 in, 2 out]
        n92 = local read "F(z)"() -> (w156:cluster{"Data":dbl[], "Data":dbl[]}[])
        n93 = Index Array(array=w156) -> (element=w155:cluster{"Data":dbl[], "Data":dbl[]})  [unwired: 1 in]
        n94 = Unbundle(w155) -> ("Data"=w134:dbl[])  [unwired: 1 out]
        n95 = for {
          tunnel: w152 -> [w175] mode=indexing
          tunnel: [w190] -> w159 mode=indexing
          tunnel: w149 -> [w172]
          tunnel: w134 -> [w185]
          shift-right: [w165] -> w153
          shift-left: w154 -> [w182]
          i -> [w173]
          n96 = call "TDMSReadWriteTraces.vi"("Channels in"=w172, "tracename"=w175) -> ("Data out"=w186:dbl[][])  [unwired: 4 in, 5 out]
          n97 = Index Array(array=w182, index (col)=0 ("index (row)")) -> (element=w184:dbl[])  [unwired: 1 in]
          n98 = call "ChangeExtension.vi"("file in"=w175) -> ("Tracenr"=w183:i32)  [unwired: 4 in, 4 out]
          n99 = Index Array(array=w186) -> (element=w164:dbl[])  [unwired: 2 in]
          n100 = Search 1D Array(1D array=w184, element=w183) -> (index of element=w167:i32)  [unwired: 1 in]
          n101 = call-poly <vilib>:"Percentiles.vi"("p"=1.0, "x array"=w164) -> ("percentile"=w171:dbl)  [unwired: 8 in, 1 out]
          n102 = Index Array(array=w182, index (row)=1, index (col)=w167) -> (element=w168:dbl)
          n103 = Add(x=w171, y=-0.1) -> (x+y=w169:dbl)
          n104 = Not Equal To 0?(x=w168) -> (x != 0?=w177:bool)
          n105 = Subtract(x=w164, y=w169) -> (x-y=w189:dbl[])
          n106 = Replace Array Subset(array=w182, new element=w169, index (row)=w167, index (col)=2 ("index (row)")) -> (w165:dbl[][])
          n107 = Bundle(w189, "Data"=w185) -> (w188:cluster{dbl[], "Data":dbl[]})  [unwired: 1 in]
          n108 = Select(t=u32 16711680, s=w177, f=u32 9868950) -> (s? t:f=w178:u32)
          n109 = call-poly <vilib>:"Percentiles.vi"("p"=5.0, "x array"=w164) -> ("percentile"=w162:dbl)  [unwired: 8 in, 1 out]
          n110 = call-poly <vilib>:"Percentiles.vi"("p"=95.0, "x array"=w164) -> ("percentile"=w191:dbl)  [unwired: 8 in, 1 out]
          n111 = property on="Select trace" class="Ring (strict)"("Value"=w173) -> ()  [unwired: 2 in, 2 out]
          n112 = Build Array(w188) -> (w187:cluster{dbl[], "Data":dbl[]}[])
          n113 = property on="F(z)" class="XYGraph (strict)"("Plot.Fill/Pt. Color"=w178) -> ()  [unwired: 2 in, 2 out]
          n114 = Subtract(x=w191, y=w162) -> (x-y=w166:dbl)
          n115 = local write "F(z)"(w187) -> ()
          n116 = Bundle(w166, w175, w169, "element"=w168) -> (w190:cluster{dbl, string, dbl, "element":dbl})  [unwired: 1 in]
        }
        n117 = Sort 1D Array(array=w159) -> (sorted array=w148:cluster{dbl, string, dbl, "element":dbl}[])
        n118 = for {
          tunnel: w148 -> [w161] mode=indexing
          tunnel: [w160] -> w151 mode=indexing
          n119 = Unbundle(w161) -> (w160:string)  [unwired: 3 out]
        }
        n120 = Index Array(array=w148) -> (element=w147:cluster{dbl, string, dbl, "element":dbl})  [unwired: 1 in]
        n121 = Unbundle(w147) -> (w146:string, w139:dbl, "element"=w141:dbl)  [unwired: 1 out]
        n122 = call "TDMSReadWriteTraces.vi"("Channels in"=w149, "tracename"=w146) -> ("Data out"=w137:dbl[][])  [unwired: 4 in, 5 out]
        n123 = Not Equal To 0?(x=w141) -> (x != 0?=w145:bool)
        n124 = Index Array(array=w137, index (row)=0) -> (element=w140:dbl[])  [unwired: 1 in]
        n125 = Select(t=u32 16711680, s=w145, f=u32 9868950) -> (s? t:f=w144:u32)
        n126 = Subtract(x=w140, y=w139) -> (x-y=w135:dbl[])
        n127 = property on="Select trace" class="Ring (strict)"("Strings []"=w151, "Value"=0 ("index (row)")) -> (error out=w157:errorcluster)  [unwired: 2 in, 1 out]
        n128 = Bundle(w135, "Data"=w134) -> (w136:cluster{dbl[], "Data":dbl[]})  [unwired: 1 in]
        n129 = property on="F(z)" class="XYGraph (strict)"("Plot.Fill/Pt. Color"=w144) -> ()  [unwired: 2 in, 2 out]
        n130 = Build Array(w136) -> (w133:cluster{dbl[], "Data":dbl[]}[])
        n131 = local write "F(z)"(w133) -> ()
        n132 = call <vilib>:"Unset Busy.vi"("error in (no error)"=w157) -> ()  [unwired: 10 in, 1 out]
      }
      event "Deselect all": Value Change {
        w197 = 1 ("disabled index (col)")
        n133 = event-data() -> ()  [unwired: 1 in, 6 out]
        n134 = Index Array(array=w198, index (col)=w197) -> (element=w199:dbl[])  [unwired: 1 in]
        n135 = Multiply(x=w199, y=0.0) -> (x*y=w196:dbl[])
        n136 = Replace Array Subset(array=w198, new element=w196, index (col)=w197) -> (w195:dbl[][])  [unwired: 1 in]
        n137 = property on="F(z)" class="XYGraph (strict)"("Plot.Fill/Pt. Color"=u32 9868950) -> ()  [unwired: 2 in, 2 out]
      }
      event "OK": Value Change {
        n138 = event-data() -> ()  [unwired: 1 in, 5 out]
        n139 = property on="Select trace" class="Ring (strict)"() -> ("Strings []"=w208:string[])  [unwired: 2 in, 2 out]
        n140 = Index Array(array=w208) -> (element=w210:string)  [unwired: 1 in]
        n141 = call "DatReadColumn.vi"("Names"=string[] ["Trace"], "tracename"=w210) -> ("Values out"=w209:dbl[][])  [unwired: 5 in, 2 out]
        n142 = Index Array(array=w201, index (col)=0 ("disabled index (col)")) -> (element=w202:dbl[])  [unwired: 1 in]
        n143 = for {
          tunnel: w209 -> [w229]
          tunnel: w208 -> [w214] mode=indexing
          shift-right: [w224] -> w205
          shift-left: string[] [] -> [w225]
          tunnel: w202 -> [w220]
          tunnel: w201 -> [w217]
          n144 = call "ChangeExtension.vi"("file in"=w214) -> ("Tracenr"=w219:i32)  [unwired: 4 in, 4 out]
          n145 = Search 1D Array(1D array=w220, element=w219) -> (index of element=w218:i32)  [unwired: 1 in]
          n146 = Index Array(array=w217, index (row)=w218) -> (element=w216:dbl[])  [unwired: 1 in]
          n147 = Index Array(array=w229, index (col)=0 ("disabled index (col)")) -> (element=w222:dbl[])  [unwired: 1 in]
          n148 = Index Array(array=w216, index=1) -> (element=w215:dbl)
          n149 = Index Array(array=w216, index=0 ("disabled index (col)")) -> (element=w223:dbl)
          n150 = Search 1D Array(1D array=w222, element=w223) -> (index of element=w221:i32)  [unwired: 1 in]
          n151 = case shown="1, Default" w221 {
            tunnel: w214 -> [w240 w247]
            tunnel: w216 -> [_ w244]
            tunnel: [w240 w242] -> w226
            tunnel: w223 -> [_ _]
            frame -1 {
            }
            frame 1, Default {
              n152 = Index Array(array=w244, index=1) -> (element=w243:dbl)
              n153 = Build Array(w243) -> (w246:dbl[])
              n154 = call "DatSaveParams.vi"("Values"=w246, "Names"=string[] ["Selected"], "tracename"=w247) -> ("tracename out"=w242:string)  [unwired: 5 in, 1 out]
            }
          }
          n155 = case shown="1" w215 {
            tunnel: w226 -> [_ w236]
            tunnel: w216 -> [_ w239]
            tunnel: w225 -> [w231 w235]
            tunnel: [w231 w234] -> w224
            frame 0, Default {
            }
            frame 1 {
              n156 = Delete From Array(array=w239, index=0) -> (array with subset deleted=w237:dbl[])  [unwired: 1 in, 1 out]
              n157 = call "DatSaveParams.vi"("Values"=w237, "Names"=string[] ["Selected", "Z0 (um)"], "tracename"=w236) -> ("tracename out"=w233:string)  [unwired: 5 in, 1 out]
              n158 = Build Array (concatenate)(w235, w233) -> (w234:string[])
            }
          }
        }
        n159 = Sort 1D Array(array=w205) -> (sorted array=→"Selected traces":string[])
        n160 = Array Size(array=w205) -> (size(s)=w212:i32)
        n161 = Less Or Equal To 0?(x=w212) -> (x <= 0?=→"No files":bool)
      }
      event "Cancel": Value Change {
        n162 = event-data() -> ()  [unwired: 1 in, 6 out]
        n163 = local write "Selected traces"(string[] [] ("Files")) -> ()
        n164 = local write "No files"("Cancel") -> ()
      }
    }
  }
